vi "Data set to SVM problem.vi"(8 "Error In":errorcluster, 10 "Data set":dbl[][](array[numeric])) -> (0 "Error Out":errorcluster, 2 "Problem out":T1)   [LabVIEW 2016]
doc: "Convert 2D input array in SVM problem format (see LIBSVM documentation for more details).\n2D input array has to be structured like this:\n\nClass label - feature 1 - feature 2 - ..... - feature N"
uses:
  <userlib>/LVLibSVM/LibSVM Sparse/Wrapper API/Controls/svm_problem.ctl
  <userlib>/LVLibSVM/LibSVM Sparse/Wrapper API/Controls/svm_node.ctl
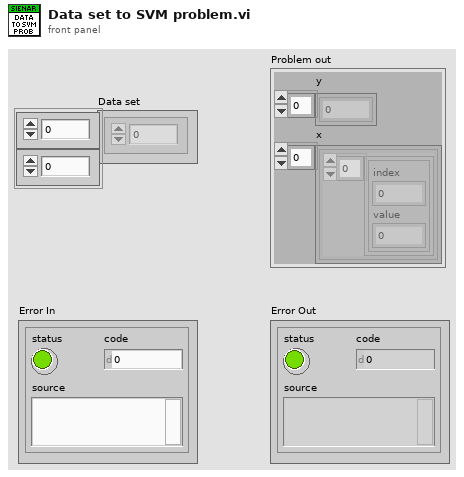
[diagram p1: front panel]
types:
  T1 = typedef "svm_problem.ctl" = cluster{"y":dbl[], "x":cluster{T2[]}[]}
  T2 = typedef "svm_node.ctl" = cluster{"index":i32, "value":dbl}
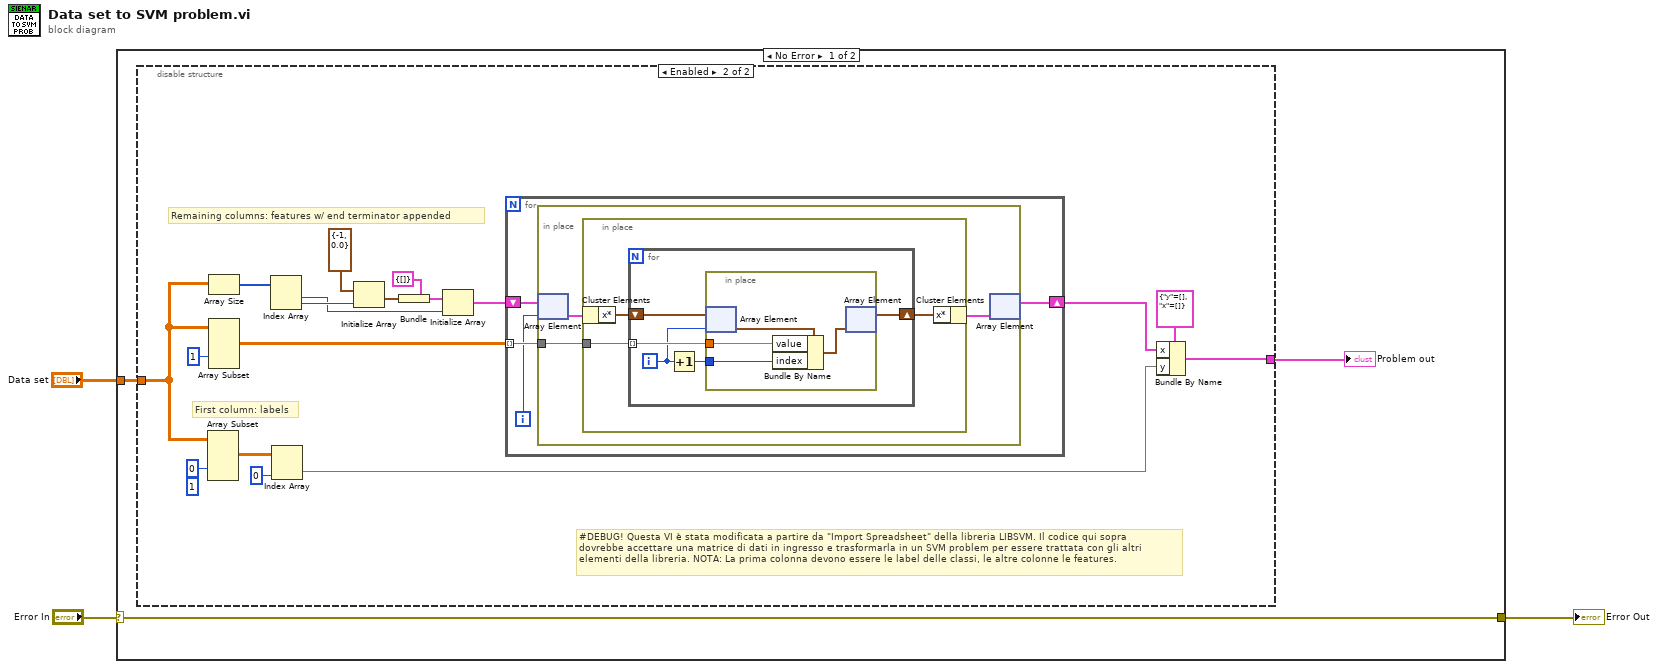
[diagram p0: block diagram]
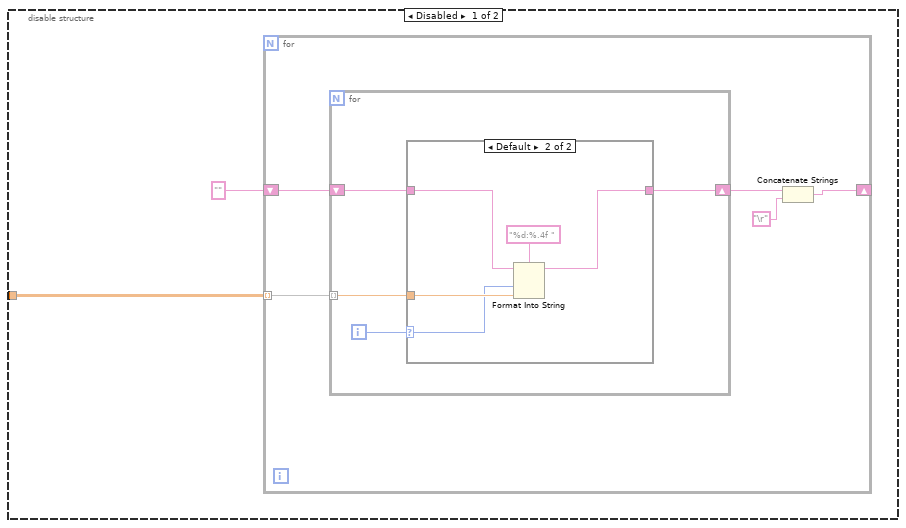
[diagram p2: hidden frame]
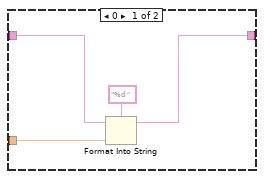
[diagram p3: hidden frame]
diagram:
  n1 = case shown="No Error" "Error In" {
    selector: "Error In" -> [w6 w65]
    tunnel: [w6 w65] -> w2
    tunnel: "Data set" -> [w5 _]
    frame No Error {
      n2 = disable-structure shown="Enabled" {
        disable-tunnel: w5 -> [w9 w29]
        disable-tunnel: [_ w28] -> w4
        frame Disabled {
          n3 = for {
            tunnel: w9 -> [w14] mode=indexing
            shift-right: [w11] -> w7
            shift-left: "" -> [w10]
            n4 = for {
              tunnel: w14 -> [w17] mode=indexing
              shift-right: [w16] -> w13
              shift-left: w10 -> [w15]
              i -> [w18]
              n5 = case shown="Default" w18 {
                selector: w18 -> [_ w23]
                tunnel: w17 -> [w21 w24]
                tunnel: [w19 w26] -> w16
                tunnel: w15 -> [w20 w25]
                frame 0 {
                  n6 = Format Into String(format string="%d ", initial string=w20, w21) -> (resulting string=w19:string)  [unwired: 1 in, 1 out]
                }
                frame Default {
                  n7 = Format Into String(format string="%d:%.4f ", initial string=w25, w23, w24) -> (resulting string=w26:string)  [unwired: 1 in, 1 out]
                }
              }
            }
            n8 = Concatenate Strings(w13, "\r") -> (w11:string)
          }
        }
        frame Enabled {
          (unwired) 1 ("length")
          # "#DEBUG! Questa VI è stata modificata a partire da \"Import Spreadsheet\" della libreria LIBSVM. Il codice qui sopra\ndovrebbe accettare una matrice di dati in ingresso e trasformarla in un SVM problem per essere trattata con gli altri\nelementi della libreria. NOTA: La prima colonna devono essere le label delle classi, le altre colonne le features."
          # "Remaining columns: features w/ end terminator appended"
          # "First column: labels"
          n9 = Array Subset(array=w29, index (col)=0 ("index")) -> (w41:dbl[][])  [unwired: 3 in]
          n10 = Array Size(array=w29) -> (size(s)=w38:i32[])
          n11 = Array Subset(array=w29, index (col)=1 ("index")) -> (w31:dbl[][])  [unwired: 3 in]
          n12 = Index Array(array=w38) -> (element #1=w34:i32, element #2=w37:i32)  [unwired: 2 in]
          n13 = Index Array(array=w41, index (col)=0 ("disabled index (col)")) -> (element=w39:dbl[])  [unwired: 1 in]
          n14 = Initialize Array(T2 {"index"=-1, "value"=0.0} ("svm_node"), w37) -> (w36:T2[])
          n15 = Bundle(cluster=cluster{"x*":T2[]} {"x*"=[]}, "x*"=w36) -> (w35:cluster{"x*":T2[]})
          n16 = Initialize Array(w35, w34) -> (w33:cluster{"x*":T2[]}[])
          n17 = for {
            tunnel: w31 -> [w49] mode=indexing
            shift-right: [w46] -> w42
            shift-left: w33 -> [w48]
            i -> [w47]
            n18 = in-place {
              in-place-border: w49 -> [w52]
              n19 = in-place-array #1(w48, w47) -> (w51:cluster{"x*":T2[]})
              n20 = in-place {
                in-place-border: w52 -> [w55]
                n21 = in-place-cluster #2(w51) -> ("x*"=w54:T2[])
                n22 = for {
                  tunnel: w55 -> [w60] mode=indexing
                  shift-right: [w56] -> w53
                  shift-left: w54 -> [w57]
                  i -> [w58]
                  n23 = Increment(x=w58) -> (x+1=w59:i32)
                  n24 = in-place {
                    in-place-border: w60 -> [w64]
                    in-place-border: w59 -> [w63]
                    n25 = in-place-array #3(w57, w58) -> (w62:T2)
                    n26 = Bundle By Name(cluster=w62, "value"=w64, "index"=w63) -> (w61:T2)
                    n27 = in-place-array #3(w61) -> (w56:T2[])  [unwired: 1 out]
                  }
                }
                n28 = in-place-cluster #2("x*"=w53) -> (w50:cluster{"x*":T2[]})
              }
              n29 = in-place-array #1(w50) -> (w46:cluster{"x*":T2[]}[])  [unwired: 1 out]
            }
          }
          n30 = Bundle By Name(cluster=T1 {"y"=[], "x"=[]} ("Problem"), "x"=w42, "y"=w39) -> (w28:T1)
        }
      }
      "Problem out" <- w4
    }
    frame Error {
    }
  }
  "Error Out" <- w2
